vi "Video_GetPalette.vi"() -> (3 "Palette":u32[](array[colorbox]))   [LabVIEW 2020]
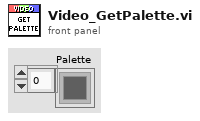
[diagram p1: front panel]
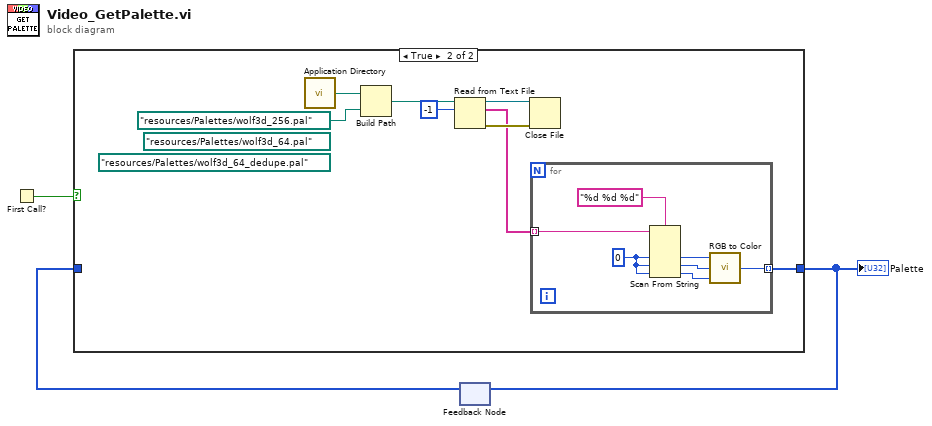
[diagram p0: block diagram]
diagram:
  n1 = First Call?() -> (First Call?: T/F=w3:bool)
  n2 = feedback #1() -> (w1:u32[])  [unwired: 1 in]
  n3 = case shown="True" w3 {
    tunnel: [w4 w6] -> w2
    tunnel: w1 -> [w4 _]
    frame False {
    }
    frame True {
      (unwired) path "resources/Palettes/wolf3d_64_dedupe.pal"
      (unwired) path "resources/Palettes/wolf3d_64.pal"
      n4 = call <vilib>:"Application Directory.vi"() -> ("Application Directory"=w12:path)
      n5 = Build Path(base path=w12, name or relative path=path "resources/Palettes/wolf3d_256.pal") -> (appended path=w11:path)
      n6 = Read from Text File(file (use dialog)=w11, count=-1) -> (refnum out=w9:refnum<file>, text=w7:string[], error out=w8:errorcluster)  [unwired: 2 in, 1 out]
      n7 = Close File(refnum=w9, error in=w8) -> ()  [unwired: 2 out]
      n8 = for {
        tunnel: w7 -> [w18] mode=indexing
        tunnel: [w13] -> w6 mode=indexing
        w16 = u8 0 ("default value 1")
        n9 = Scan From String(format string="%d %d %d", input string=w18, default 1=w16, default 2=w16, default 3=w16) -> (output 1=w17:u8, output 2=w15:u8, output 3=w14:u8)  [unwired: 2 in, 3 out]
        n10 = call <vilib>:"RGB to Color.vi"("B"=w14, "G"=w15, "R"=w17) -> ("Color"=w13:u32)
      }
    }
  }
  "Palette" <- w2
  n11 = feedback-in #1(w2) -> ()
